vi "Statically-sized Cluster.vi"   [LabVIEW 2020, in "Memory Manager Tests.lvlib" / "Malleable Type Tests.lvclass"]
uses:
  Malleable Type Tests.lvclass
  6a220805-c7e9-49bf-aec1-35ff7729ed96.vi
  Source/Classes/Pointer/Check Null Pointer.vi
  Source/Classes/Pointer/Get Size.vi
  Source/Classes/Pointer/Get Address.vi
  Source/Classes/Pointer/Pointer.lvclass
  Malleable Type Tests.lvclass/Malleable Type Tests.ctl
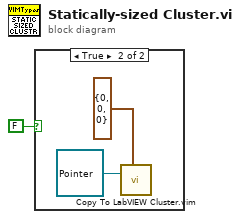
[diagram p0: block diagram]
diagram:
  n1 = case shown="True" FALSE {
    frame False {
    }
    frame True {
      n2 = call "Copy To LabVIEW Cluster.vim"("Type"=cluster{i32, i32, i32} {0, 0, 0}, "Pointer in"=refnum<class "Pointer.lvclass"> refnum) -> ()  [unwired: 7 in, 3 out]
    }
  }
